vi "FL Plot Variable.vi"(5 "variable index":i32, 7 "input/output":T13 items=["Input", "Output"], 8 "error in (no error)":errorcluster, 10 "graph refnum":refnum<vi>, 11 "fuzzy system in":T1 {"user MF interpolating polynomials"."coa_x(y) coeff" format="%.4g"; "user MF interpolating polynomials"."Area(y) coeff" format="%.4g"; "user MF interpolating polynomials"."X(y) coeff" format="%.4g"; "user MF interpolating polynomials"."Y(x) coeff" format="%.4g"; "user MF interpolating polynomials"."Y" format="%.4g"; "user MF interpolating polynomials"."X" format="%.4g"; "defuzzification method" items=["Center of Area", "Modified Center of Area", "Center of Sums", "Center of Maximum", "Mean of Maximum"]; "rules"."consequents"."Var Index" min=0; "rules"."consequents"."Cond" items=["=", "!="]; "rules"."consequents"."MF Index" min=0; "rules"."antecedents"."Var Index" min=0; "rules"."antecedents"."Cond" items=["=", "!="]; "rules"."antecedents"."MF Index" min=0; "rules"."consequent implication" items=["Minimum", "Product"]; "rules"."antecedent connective" items=["AND (Minimum)", "AND (Product)", "OR (Maximum)", "OR (Probabilistic)"]; "output variables"."MFs"."shape" items=["Triangle", "Trapezoid", "Singleton", "Sigmoid", "Gaussian", "User-Defined"]; "input variables"."MFs"."shape" items=["Triangle", "Trapezoid", "Singleton", "Sigmoid", "Gaussian", "User-Defined"]}) -> (0 "error out":errorcluster, 2 "membership functions plot":cluster{cluster{"Xi":dbl, "Yi":dbl}[]}[](graph), 3 "fuzzy system out":T1 {"user MF interpolating polynomials"."coa_x(y) coeff" format="%.4g"; "user MF interpolating polynomials"."Area(y) coeff" format="%.4g"; "user MF interpolating polynomials"."X(y) coeff" format="%.4g"; "user MF interpolating polynomials"."Y(x) coeff" format="%.4g"; "user MF interpolating polynomials"."Y" format="%.4g"; "user MF interpolating polynomials"."X" format="%.4g"; "defuzzification method" items=["Center of Area", "Modified Center of Area", "Center of Sums", "Center of Maximum", "Mean of Maximum"]; "rules"."consequents"."Var Index" min=0; "rules"."consequents"."Cond" items=["=", "!="]; "rules"."consequents"."MF Index" min=0; "rules"."antecedents"."Var Index" min=0; "rules"."antecedents"."Cond" items=["=", "!="]; "rules"."antecedents"."MF Index" min=0; "rules"."consequent implication" items=["Minimum", "Product"]; "rules"."antecedent connective" items=["AND (Minimum)", "AND (Product)", "OR (Maximum)", "OR (Probabilistic)"]; "output variables"."MFs"."shape" items=["Triangle", "Trapezoid", "Singleton", "Sigmoid", "Gaussian", "User-Defined"]; "input variables"."MFs"."shape" items=["Triangle", "Trapezoid", "Singleton", "Sigmoid", "Gaussian", "User-Defined"]})   [LabVIEW 2017, in "NI_Fuzzy_Logic_API.lvlib"]
doc: "Plots a specific input or output variable that is in a fuzzy system with the membership functions of that variable."
uses:
  <vilib>/addons/Fuzzy Logic/NI_Fuzzy_Logic_API.lvlib
  <vilib>/addons/Fuzzy Logic/TypeDefs/FL System.ctl
  <vilib>/addons/Fuzzy Logic/TypeDefs/FL Variable.ctl
  <vilib>/addons/Fuzzy Logic/TypeDefs/FL Membership Function.ctl
  <vilib>/addons/Fuzzy Logic/TypeDefs/FL Membership Function Shape.ctl
  <vilib>/addons/Fuzzy Logic/TypeDefs/FL Rule.ctl
  <vilib>/addons/Fuzzy Logic/TypeDefs/FL Antecedent.ctl
  <vilib>/addons/Fuzzy Logic/TypeDefs/FL Modifier.ctl
  <vilib>/addons/Fuzzy Logic/TypeDefs/FL Antecedent Connective.ctl
  <vilib>/addons/Fuzzy Logic/TypeDefs/FL Consequent.ctl
  <vilib>/addons/Fuzzy Logic/TypeDefs/FL Consequent Implication.ctl
  <vilib>/addons/Fuzzy Logic/TypeDefs/FL Defuzzification.ctl
  <vilib>/addons/Fuzzy Logic/TypeDefs/FL Interpolating polynomials.ctl
  <vilib>/addons/Fuzzy Logic/TypeDefs/FL Input_Output.ctl
  <vilib>/Analysis/1siggen.llb/Ramp Pattern by Samples.vi
  <vilib>/Analysis/NI_AALBase.lvlib
panel:
  out "graph error":errorcluster
  # "IF"
  # "THEN"
  # "IF"
  # "THEN"
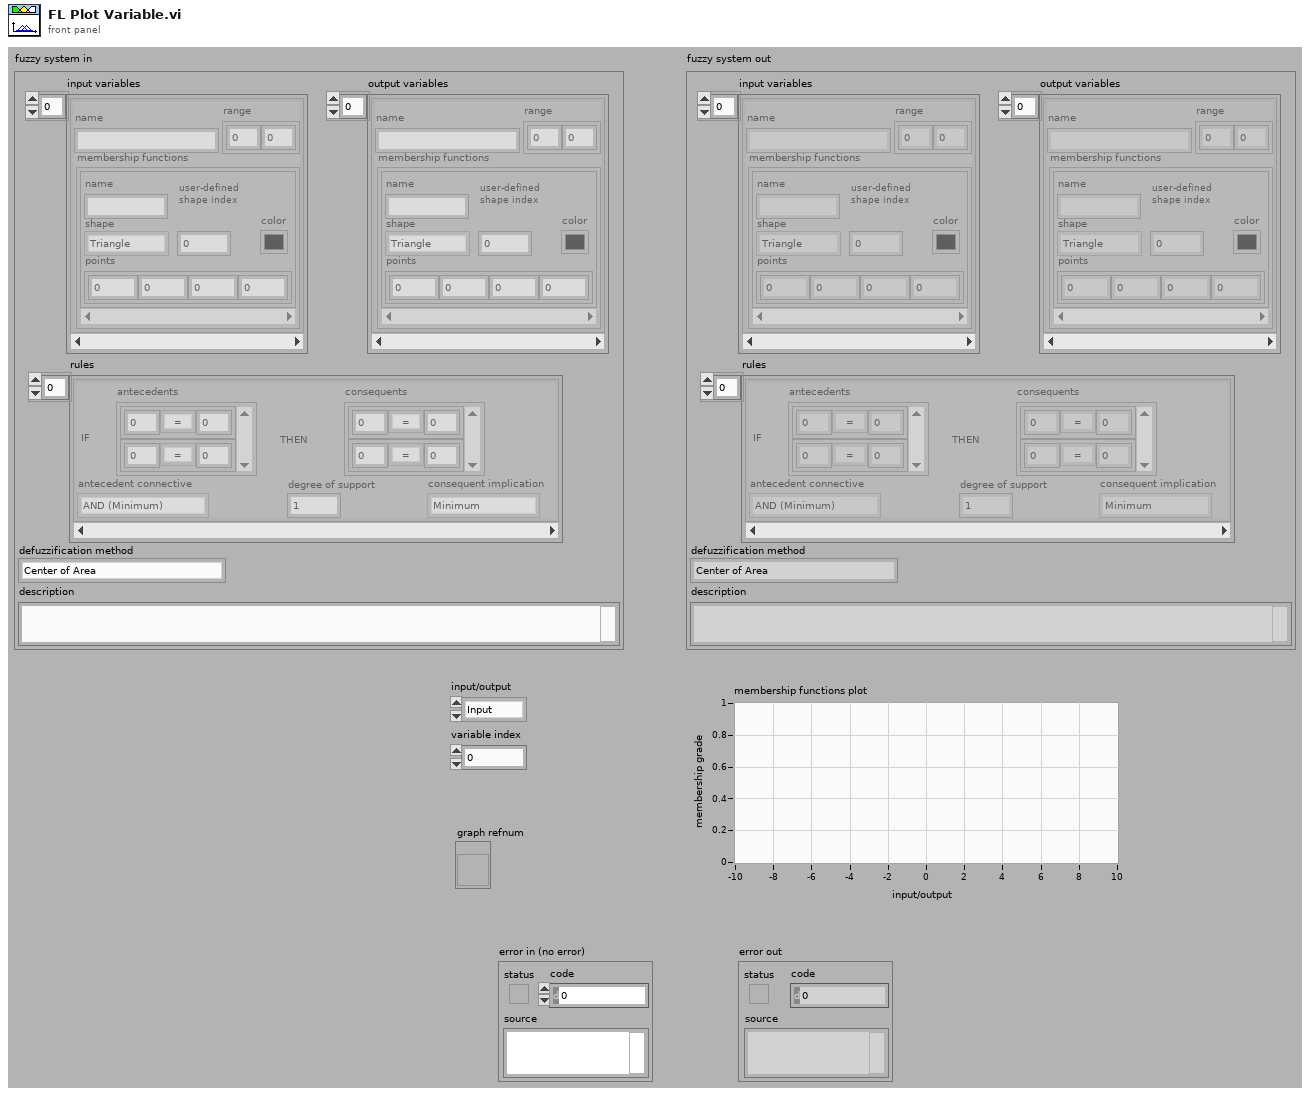
[diagram p1: front panel]
types:
  T1 = typedef "NI_Fuzzy_Logic_API.lvlib/FL System.ctl" = cluster{"input variables":T2[], "output variables":T2[], "rules":T5[], "defuzzification method":T11, "description":string, "user MF interpolating polynomials":T12[]}
  T2 = typedef "NI_Fuzzy_Logic_API.lvlib/FL Variable.ctl" = cluster{"name":string, "range":dbl[], "MFs":T3[]}
  T3 = typedef "NI_Fuzzy_Logic_API.lvlib/FL Membership Function.ctl" = cluster{"name":string, "shape":T4, "points":dbl[], "color":u32, "user-defined shape index":i32}
  T4 = typedef "NI_Fuzzy_Logic_API.lvlib/FL Membership Function Shape.ctl" = u16
  T5 = typedef "NI_Fuzzy_Logic_API.lvlib/FL Rule.ctl" = cluster{"antecedents":T6[], "antecedent connective":T8, "consequents":T9[], "consequent implication":T10, "degree of support":dbl}
  T6 = typedef "NI_Fuzzy_Logic_API.lvlib/FL Antecedent.ctl" = cluster{"Var Index":i32, "MF Index":i32, "Cond":T7}
  T7 = typedef "NI_Fuzzy_Logic_API.lvlib/FL Modifier.ctl" = u16
  T8 = typedef "NI_Fuzzy_Logic_API.lvlib/FL Antecedent Connective.ctl" = u16
  T9 = typedef "NI_Fuzzy_Logic_API.lvlib/FL Consequent.ctl" = cluster{"Var Index":i32, "MF Index":i32, "Cond":T7}
  T10 = typedef "NI_Fuzzy_Logic_API.lvlib/FL Consequent Implication.ctl" = u16
  T11 = typedef "NI_Fuzzy_Logic_API.lvlib/FL Defuzzification.ctl" = u16
  T12 = typedef "NI_Fuzzy_Logic_API.lvlib/FL Interpolating polynomials.ctl" = cluster{"X":dbl[], "Y":dbl[], "Y(x) coeff":dbl[][], "X(y) coeff":dbl[][], "Area(y) coeff":dbl[][], "coa_x(y) coeff":dbl[][]}
  T13 = typedef "NI_Fuzzy_Logic_API.lvlib/FL Input_Output.ctl" = u16
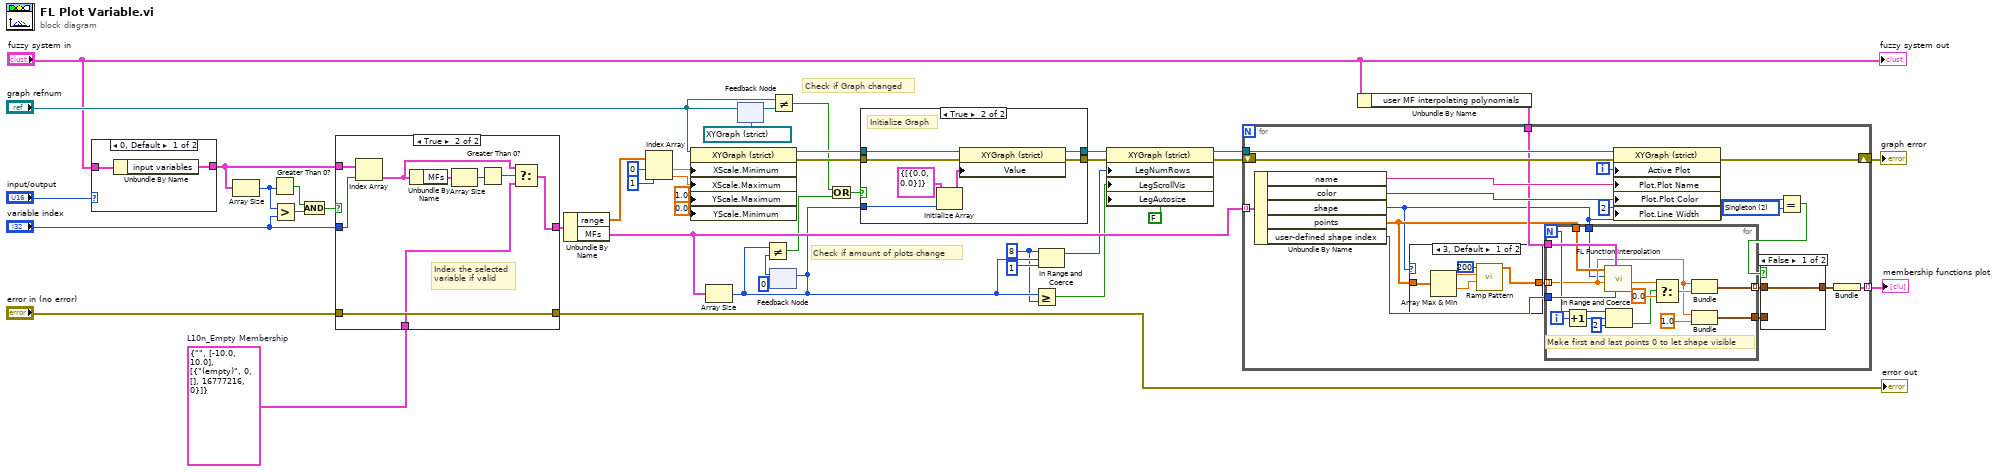
[diagram p0: block diagram]
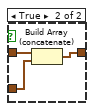
[diagram p2: hidden frame]
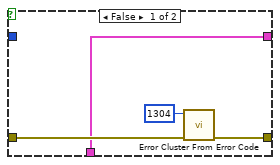
[diagram p4: hidden frame]
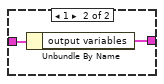
[diagram p5: hidden frame]
diagram:
  w1 = T2 {"name"="", "range"=[-10.0, 10.0], "MFs"=[{"name"="(empty)", "shape"=0, "points"=[], "color"=16777216, "user-defined shape index"=0}]}  # L10n_Empty Membership
  w9 = 8 ("upper limit")
  # "Check if Graph changed"
  # "Check if amount of plots change"
  n1 = case shown="0, Default" "input/output" {
    tunnel: "fuzzy system in" -> [w45 w47]
    tunnel: [w44 w46] -> w30
    frame 0, Default {
      n2 = Unbundle By Name(w45) -> ("input variables"=w44:T2[])
    }
    frame 1 {
      n3 = Unbundle By Name(w47) -> ("output variables"=w46:T2[])
    }
  }
  n4 = Array Size(array=w30) -> (size(s)=w33:i32)
  n5 = Greater Than 0?(x=w33) -> (x > 0?=w32:bool)
  n6 = Greater?(x=w33, y="variable index") -> (0:w34:bool)
  n7 = And(x=w32, y=w34) -> (x .and. y?=w31:bool)
  n8 = case shown="True" w31 {
    tunnel: [w48 w53] -> w27
    tunnel: w30 -> [_ w60]
    tunnel: "variable index" -> [_ w59]
    tunnel: [w50 w58] -> w19
    tunnel: "error in (no error)" -> [w51 w58]
    tunnel: w1 -> [w48 w52]
    frame False {
      n9 = call <vilib>:"Error Cluster From Error Code.vi"("error in (no error)"=w51, "error code (0)"=1304) -> ("error out"=w50:errorcluster)  [unwired: 1 in, 6 out]
    }
    frame True {
      # "Index the selected\nvariable if valid"
      n10 = Index Array(array=w60, index=w59) -> (element=w54:T2)
      n11 = Unbundle By Name(w54) -> ("MFs"=w56:T3[])
      n12 = Array Size(array=w56) -> (size(s)=w57:i32)
      n13 = Greater Than 0?(x=w57) -> (x > 0?=w55:bool)
      n14 = Select(t=w54, s=w55, f=w52) -> (s? t:f=w53:T2)
    }
  }
  "error out" <- w19
  n15 = Unbundle By Name(w27) -> ("range"=w6:dbl[], "MFs"=w39:T3[])
  n16 = Index Array(array=w6, index #1=0 ("index"), index #2=1 ("index")) -> (element #1=w3:dbl, element #2=w2:dbl)
  n17 = property on="Property Node" class="XYGraph (strict)"(reference="graph refnum", "XScale.Minimum"=w3, "XScale.Maximum"=w2, "YScale.Maximum"=1.0 ("Y Scale.Range:Maximum"), "YScale.Minimum"=0.0 ("Y Scale.Range:Minimum")) -> (reference out=w42:refnum<vi>, error out=w26:errorcluster)  [unwired: 1 in]
  n18 = Array Size(array=w39) -> (size(s)=w22:i32)
  n19 = feedback-in #1("graph refnum") -> ()
  n20 = feedback #1(refnum<vi> refnum ("Graph Refnum")) -> (w16:refnum<vi>)
  n21 = feedback-in #2(w22) -> ()
  n22 = feedback #2(0) -> (w23:i32)
  n23 = Not Equal?(x=w22, y=w23) -> (x != y?=w21:bool)
  n24 = Not Equal?(x="graph refnum", y=w16) -> (x != y?=w14:bool)
  n25 = Or(x=w14, y=w21) -> (x .or. y?=w20:bool)
  n26 = case shown="True" w20 {
    tunnel: w42 -> [w62 w69]
    tunnel: [w62 w64] -> w40
    tunnel: w26 -> [w61 w68]
    tunnel: [w61 w63] -> w25
    tunnel: w22 -> [_ w65]
    frame False {
    }
    frame True {
      # "Initialize Graph"
      n27 = Initialize Array(cluster{"Function Graph":cluster{dbl, dbl}[]} {"Function Graph"=[{0.0, 0.0}]}, w65) -> (w66:cluster{"Function Graph":cluster{dbl, dbl}[]}[])
      n28 = property on="Property Node" class="XYGraph (strict)"(reference=w69, error in=w68, "Value"=w66) -> (reference out=w64:refnum<vi>, error out=w63:errorcluster)
    }
  }
  n29 = Greater Or Equal?(x=w22, y=w9) -> (x >= y?=w36:bool)
  n30 = In Range and Coerce(upper limit=w9, x=w22, lower limit=1) -> (coerced(x)=w38:i32)  [unwired: 1 out]
  n31 = property on="Property Node" class="XYGraph (strict)"(reference=w40, error in=w25, "LegNumRows"=w38, "LegScrollVis"=w36, "LegAutosize"=FALSE ("Legend:Autosize")) -> (reference out=w41:refnum<vi>, error out=w24:errorcluster)
  n32 = Unbundle By Name("fuzzy system in") -> ("user MF interpolating polynomials"=w8:T12[])
  n33 = for {
    tunnel: w39 -> [w86] mode=indexing
    tunnel: w41 -> [w84]
    tunnel: [w83] -> w43 mode=indexing
    shift-right: [w81] -> w18
    shift-left: w24 -> [w82]
    tunnel: w8 -> [w80]
    i -> [w85]
    w75 = T4 2 items=["Triangle", "Trapezoid", "Singleton", "Sigmoid", "Gaussian", "User-Defined"] ("y")
    n34 = Unbundle By Name(w86) -> ("name"=w87:string, "color"=w88:u32, "shape"=w74:T4, "points"=w78:dbl[], "user-defined shape index"=w76:i32)
    n35 = case shown="3, Default" w74 {
      tunnel: [w93 w98] -> w79
      tunnel: w78 -> [w95 w98]
      frame 3, Default {
        n36 = Array Max & Min(array=w95) -> (max value=w97:dbl, min value=w96:dbl)  [unwired: 2 out]
        n37 = call-poly <vilib>:"Ramp Pattern.vi"("start"=w96, "end"=w97, "samples"=200) -> ("Ramp Pattern"=w93:dbl[])  [unwired: 7 in, 1 out]
      }
      frame 0..2 {
      }
    }
    n38 = for {
      N -> [w107]
      tunnel: w80 -> [w114]
      tunnel: w79 -> [w103] mode=indexing
      tunnel: [w100] -> w72 mode=indexing
      tunnel: w74 -> [w101]
      tunnel: w78 -> [w113]
      tunnel: w76 -> [w112]
      tunnel: [w99] -> w70
      i -> [w106]
      # "Make first and last points 0 to let shape visible"
      n39 = Increment(x=w106) -> (x+1=w105:i32)
      n40 = call <vilib>:"FL Function Interpolation.vi"("user-defined \nshape index"=w112, "user MF interpolating polynomials"=w114, "Input Data"=w103, "shape"=w101, "Points"=w113) -> ("Membership"=w109:dbl)  [unwired: 1 in, 5 out]
      n41 = In Range and Coerce(upper limit=w107, x=w105, lower limit=2) -> (In Range?=w104:bool)  [unwired: 1 out]
      n42 = Select(t=w109, s=w104, f=0.0) -> (s? t:f=w110:dbl)
      n43 = Bundle("Numeric"=w103, "f"=w110) -> (w100:cluster{"Numeric":dbl, "f":dbl})  [unwired: 1 out]
      n44 = Bundle("Numeric"=w103, "f"=1.0) -> (w99:cluster{"Numeric":dbl, "f":dbl})  [unwired: 1 out]
    }
    n45 = property on="Property Node" class="XYGraph (strict)"(reference=w84, error in=w82, "Active Plot"=w85, "Plot.Plot Name"=w87, "Plot.Plot Color"=w88, "Plot.Line Width"=u8 2) -> (error out=w81:errorcluster)  [unwired: 1 out]
    n46 = Equal?(x=w74, y=w75) -> (x = y?=w73:bool)
    n47 = case shown="False" w73 {
      tunnel: w72 -> [w89 w92]
      tunnel: [w89 w90] -> w71
      tunnel: w70 -> [_ w91]
      frame False {
      }
      frame True {
        n48 = Build Array (concatenate)(w92, w91) -> (w90:cluster{"Numeric":dbl, "f":dbl}[])
      }
    }
    n49 = Bundle(w71) -> (w83:cluster{cluster{"Numeric":dbl, "f":dbl}[]})  [unwired: 1 in]
  }
  "membership functions plot" <- w43
  "graph error" <- w18
  "fuzzy system out" <- "fuzzy system in"
